vi "Parse Duty Cycle from Result.vi"(8 "error in (no error)":errorcluster, 11 "ReadCommand In":refnum<class "ReadCommand.lvclass">) -> (0 "error out":errorcluster, 3 "Duty Cycle":i32 format="%.0g")   [LabVIEW 2023]
uses:
  ReadCommand/ReadCommand.lvclass
  User Defined Read/User Defined Read.lvclass
  HAF.lvlib
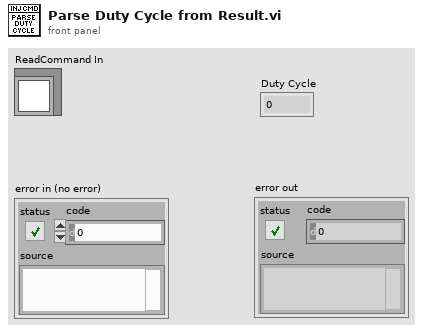
[diagram p1: front panel]
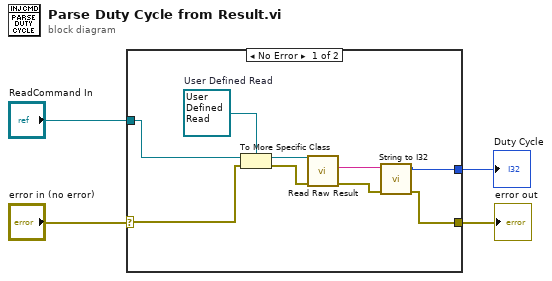
[diagram p0: block diagram]
diagram:
  n1 = case shown="No Error" "error in (no error)" {
    selector: "error in (no error)" -> [w11 w14]
    tunnel: "ReadCommand In" -> [w12 _]
    tunnel: [w6 _] -> w2
    tunnel: [w5 w14] -> w1
    frame No Error {
      w13 = refnum<class "User Defined Read.lvclass"> refnum  # User Defined Read
      n2 = To More Specific Class(target class=w13, reference=w12, error in=w11) -> (specific class reference=w10:refnum<class "User Defined Read.lvclass">, error out=w9:errorcluster)
      n3 = call-dynamic "Read Raw Result.vi"("error in (no error)"=w9, "ReadCommand in"=w10) -> ("error out"=w7:errorcluster, "Raw Result"=w8:string)  [unwired: 7 in, 1 out]
      n4 = call "String to I32.vi"("error in (no error)"=w7, "String to Convert"=w8) -> ("error out"=w5:errorcluster, "I32 Value"=w6:i32)  [unwired: 8 in]
    }
    frame Error {
    }
  }
  "error out" <- w1
  "Duty Cycle" <- w2
